vi "Circle Buffer(DBL).vi"(4 "reset(F)":bool, 5 "#Count":i32=1000, 6 "valid?(T)":bool=TRUE, 9 "Data":dbl) -> (2 "integral multiple":bool, 3 "Array":dbl[](array[numeric]))   [LabVIEW 2017]
doc: "Maintains a circular buffer of #Count doubles, writing Data into the next slot on each call and returning the whole buffer. The integral multiple output turns TRUE once the buffer has been filled a whole number of times."
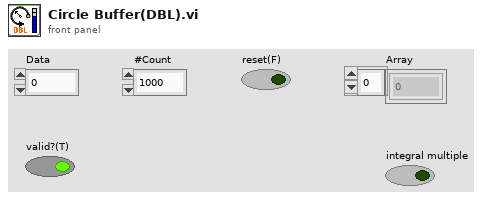
[diagram p1: front panel]
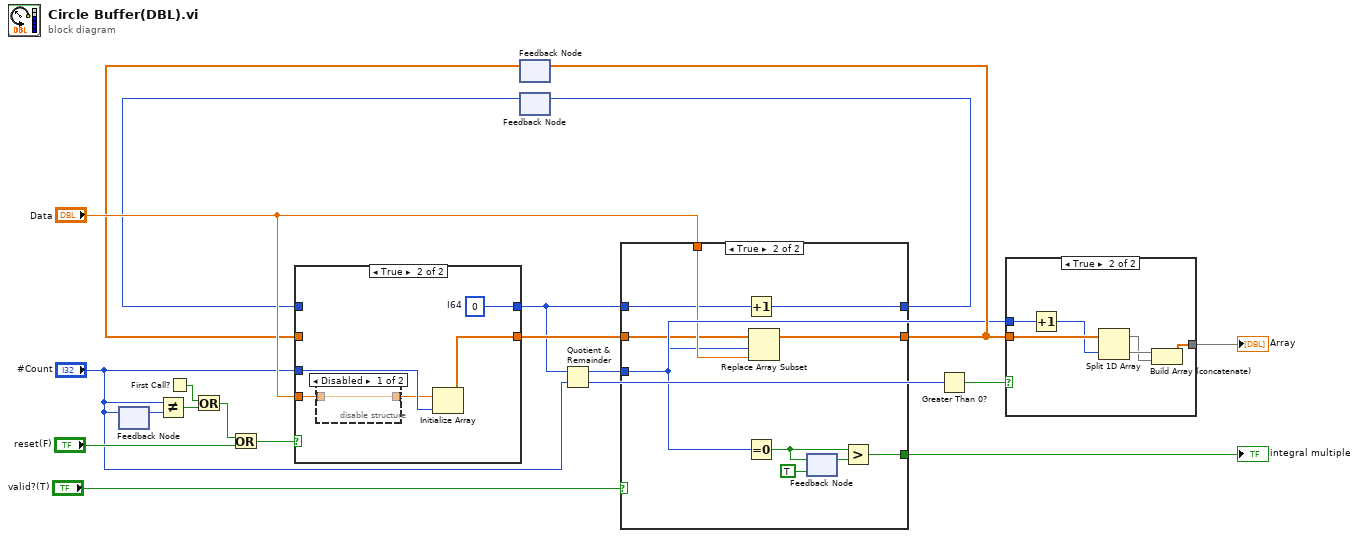
[diagram p0: block diagram]
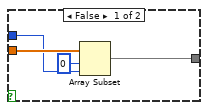
[diagram p5: hidden frame]
diagram:
  n1 = feedback #1() -> (w4:i32)  [unwired: 1 in]
  n2 = feedback-in #1("#Count") -> ()
  n3 = Not Equal?(x="#Count", y=w4) -> (x != y?=w3:bool)
  n4 = First Call?() -> (First Call?: T/F=w1:bool)
  n5 = Or(x=w1, y=w3) -> (x .or. y?=w2:bool)
  n6 = Or(x=w2, y="reset(F)") -> (x .or. y?=w7:bool)
  n7 = feedback #2() -> (w17:dbl[])  [unwired: 1 in]
  n8 = feedback #3() -> (w18:i64)  [unwired: 1 in]
  n9 = case shown="True" w7 {
    tunnel: "Data" -> [_ w25]
    tunnel: "#Count" -> [_ w27]
    tunnel: [w21 w24] -> w10
    tunnel: [w22 w23] -> w9
    tunnel: w18 -> [w22 _]
    tunnel: w17 -> [w21 _]
    frame False {
    }
    frame True {
      w23 = i64 0  # I64
      n10 = disable-structure shown="Disabled" {
        disable-tunnel: [w28 _] -> w26
        disable-tunnel: w25 -> [w28 _]
        frame Disabled {
        }
        frame Enabled {
        }
      }
      n11 = Initialize Array(w26, w27) -> (w24:dbl[])
    }
  }
  n12 = Quotient & Remainder(x=w9, y="#Count") -> (x-y*floor(x/y)=w12:i64, floor(x/y)=w8:i64)
  n13 = case shown="True" "valid?(T)" {
    tunnel: "Data" -> [_ w40]
    tunnel: [w29 w39] -> w19
    tunnel: [w30 w38] -> w16
    tunnel: w12 -> [_ w37]
    tunnel: [_ w36] -> w11
    tunnel: w10 -> [w30 w35]
    tunnel: w9 -> [w29 w34]
    frame False {
    }
    frame True {
      n14 = Increment(x=w34) -> (x+1=w39:i64)
      n15 = Equal To 0?(x=w37) -> (x = 0?=w33:bool)
      n16 = Replace Array Subset(array=w35, new element=w40, index=w37) -> (w38:dbl[])
      n17 = feedback #4(TRUE ("signal")) -> (w31:bool)
      n18 = feedback-in #4(w33) -> ()
      n19 = Greater?(x=w33, y=w31) -> (0:w36:bool)
    }
  }
  "integral multiple" <- w11
  n20 = feedback-in #2(w16) -> ()
  n21 = feedback-in #3(w19) -> ()
  n22 = Greater Than 0?(x=w8) -> (x > 0?=w15:bool)
  n23 = case shown="True" w15 {
    tunnel: w16 -> [w44 w50]
    tunnel: w12 -> [w43 w49]
    tunnel: [w41 w46] -> w14
    frame False {
      n24 = Array Subset(array=w44, index=0, length=w43) -> (w41:dbl[])
    }
    frame True {
      n25 = Increment(x=w49) -> (x+1=w45:i64)
      n26 = Split 1D Array(array=w50, index=w45) -> (first subarray=w47:dbl[], second subarray=w48:dbl[])
      n27 = Build Array (concatenate)(w48, w47) -> (w46:dbl[])
    }
  }
  "Array" <- w14
